vi "turnVelocityPlanning.vi"(4 "v_ang (rad/s)":dbl=4.0 format="%#_13g", 5 "PID gains Angles to turn":T1={"proportional gain (Kc)"=4.0, "integral time (Ti, min)"=0.0, "derivative time (Td, min)"=0.001} {"derivative time (Td, min)" format="%.3f"; "integral time (Ti, min)" format="%.10f"; "proportional gain (Kc)" format="%.3f"}, 6 "radius (mm)":dbl=140.0 format="%.2f", 7 "PID gains radius to turn":T1={"proportional gain (Kc)"=4.0, "integral time (Ti, min)"=0.0, "derivative time (Td, min)"=0.0} {"derivative time (Td, min)" format="%.3f"; "integral time (Ti, min)" format="%.3f"; "proportional gain (Kc)" format="%.3f"}, 8 "error in (no error)":errorcluster, 10 "Clockwise?":bool, 11 "Robot in":refnum<class "Robot.lvclass">) -> (0 "error out":errorcluster, 3 "Robot out":refnum<class "Robot.lvclass">)   [LabVIEW 2023, in "Robot.lvclass"]
uses:
  Robot.lvclass
  C:/Users/ebert/Desktop/roboime/SSL_AI/Object_class/Object.lvclass
  Robot.lvclass/Robot.ctl
  Object_class/Object.lvclass/Object.ctl
  <vilib>/Analysis/coordinate.llb/Wrap Angle (scalar).vi
  <vilib>/Analysis/baseanly.llb/Unit Vector (DBL).vi
  <vilib>/Analysis/coordinate.llb/2D Cartesian Coordinate Rotation (Scalar).vi
  Read dest_x.vi
  Read dest_y.vi
  Object_class/Read position(x,y).vi
  Read orientation.vi
  Write v_ang.vi
  Write v_tang.vi
  Write v_norm.vi
  <vilib>/addons/control/pid/pid.llb/PID (DBL).vi
  <vilib>/Analysis/NI_AALPro.lvlib
  <vilib>/Analysis/NI_AALBase.lvlib
  Utilities_class/Utilities.lvclass
  <vilib>/addons/control/pid/NI_PID_pid.lvlib
  <vilib>/Analysis/NI_AAL_Angle.lvlib
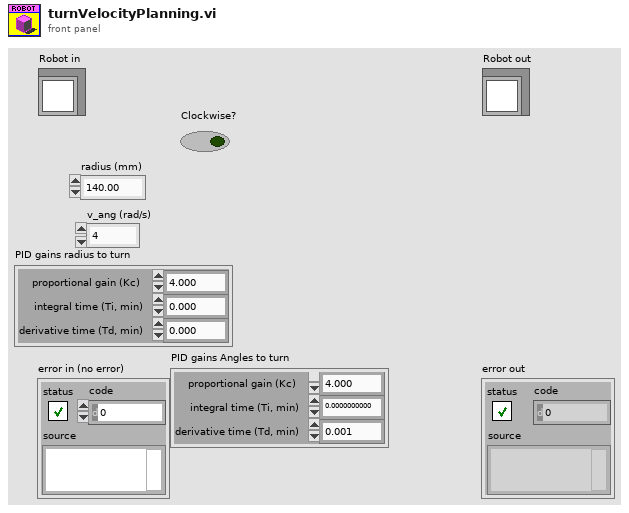
[diagram p1: front panel]
types:
  T1 = cluster{"proportional gain (Kc)":dbl, "integral time (Ti, min)":dbl, "derivative time (Td, min)":dbl}
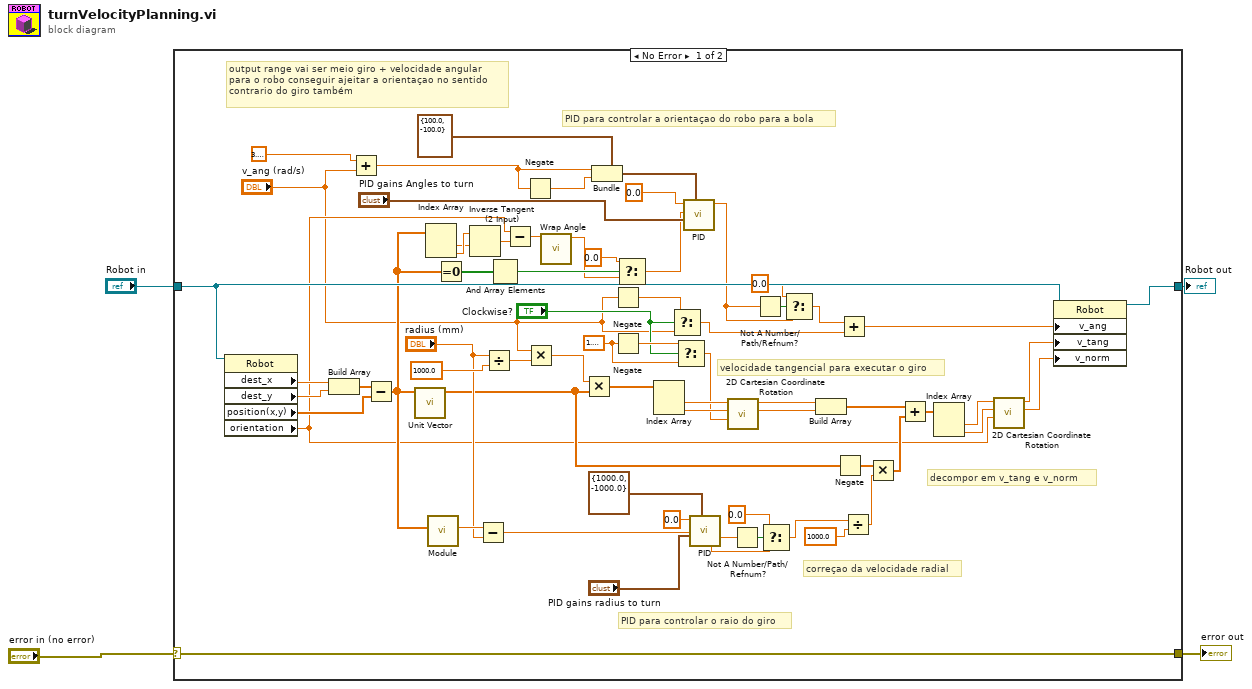
[diagram p0: block diagram]
diagram:
  n1 = case shown="No Error" "error in (no error)" {
    selector: "error in (no error)" -> [w70 w72]
    tunnel: [w70 w72] -> w3
    tunnel: [w61 w71] -> w1
    tunnel: "Robot in" -> [w62 w71]
    frame No Error {
      w27 = 1.5707963267948966
      # "correçao da velocidade radial"
      # "velocidade tangencial para executar o giro"
      # "output range vai ser meio giro + velocidade angular\npara o robo conseguir ajeitar a orientaçao no sentido\ncontrario do giro também"
      # "decompor em v_tang e v_norm"
      # "PID para controlar o raio do giro"
      # "PID para controlar a orientaçao do robo para a bola"
      n2 = property class="Robot"(reference=w62) -> ("dest_x"=w69:dbl, "dest_y"=w68:dbl, "position(x,y)"=w66:dbl[], "orientation"=w19:dbl)  [unwired: 1 in, 2 out]
      n3 = Build Array(w69, w68) -> (w67:dbl[])
      n4 = Add(x=3.141592653589793, y="v_ang (rad/s)") -> (x+y=w15:dbl)
      n5 = Subtract(x=w67, y=w66) -> (x-y=w32:dbl[])
      n6 = call-poly <vilib>:"Unit Vector.vi"("Input Vector"=w32) -> ("Unit Vector"=w43:dbl[])  [unwired: 8 in, 2 out]
      n7 = Index Array(array=w32) -> (element #1=w34:dbl, element #2=w35:dbl)  [unwired: 2 in]
      n8 = call "Module.vi"("2D vector"=w32) -> ("Modulo"=w55:dbl)  [unwired: 8 in, 2 out]
      n9 = Equal To 0?(x=w32) -> (x = 0?=w31:bool[])
      n10 = Inverse Tangent (2 Input)(1:w34, 2:w35) -> (0:w18:dbl)
      n11 = Subtract(x=w55, y="radius (mm)") -> (x-y=w53:dbl)
      n12 = Divide(x="radius (mm)", y=1000.0) -> (x/y=w59:dbl)
      n13 = And Array Elements(Boolean array=w31) -> (logical AND=w30:bool)
      n14 = Subtract(x=w19, y=w18) -> (x-y=w17:dbl)
      n15 = Negate(x=w15) -> (-x=w36:dbl)
      n16 = Multiply(x="v_ang (rad/s)", y=w59) -> (x*y=w58:dbl)
      n17 = call-poly <vilib>:"Wrap Angle.vi"("angle in"=w17) -> ("angle out"=w16:dbl)  [unwired: 9 in, 1 out]
      n18 = Multiply(x=w58, y=w43) -> (x*y=w65:dbl[])
      n19 = Bundle(cluster=cluster{"output high":dbl, "output low":dbl} {"output high"=100.0, "output low"=-100.0} ("output range"), "output high"=w15, "output low"=w36) -> (w37:cluster{"output high":dbl, "output low":dbl})
      n20 = Negate(x="v_ang (rad/s)") -> (-x=w23:dbl)
      n21 = Negate(x=w27) -> (-x=w24:dbl)
      n22 = Select(t=0.0, s=w30, f=w16) -> (s? t:f=w28:dbl)
      n23 = Index Array(array=w65) -> (element #1=w64:dbl, element #2=w63:dbl)  [unwired: 2 in]
      n24 = Select(t=w23, s="Clockwise?", f="v_ang (rad/s)") -> (s? t:f=w25:dbl)
      n25 = Select(t=w24, s="Clockwise?", f=w27) -> (s? t:f=w26:dbl)
      n26 = call-poly <vilib>:"PID.vi"("output range"=w37, "PID gains"="PID gains Angles to turn", "process variable"=w28, "setpoint"=0.0) -> ("output"=w5:dbl)  [unwired: 6 in, 1 out]
      n27 = call-poly <vilib>:"PID.vi"("output range"=cluster{"output high":dbl, "output low":dbl} {"output high"=1000.0, "output low"=-1000.0}, "PID gains"="PID gains radius to turn", "process variable"=w53, "setpoint"=0.0) -> ("output"=w11:dbl)  [unwired: 6 in, 1 out]
      n28 = call-poly <vilib>:"2D Cartesian Coordinate Rotation.vi"("theta"=w26, "y"=w63, "x"=w64) -> ("y out"=w49:dbl, "x out"=w50:dbl)  [unwired: 6 in, 1 out]
      n29 = Not A Number/Path/Refnum?(number/path/refnum=w11) -> (NaN/Path/Refnum?=w12:bool)
      n30 = Not A Number/Path/Refnum?(number/path/refnum=w5) -> (NaN/Path/Refnum?=w7:bool)
      n31 = Select(t=0.0, s=w12, f=w11) -> (s? t:f=w10:dbl)
      n32 = Select(t=0.0, s=w7, f=w5) -> (s? t:f=w6:dbl)
      n33 = Build Array(w50, w49) -> (w48:dbl[])
      n34 = Negate(x=w43) -> (-x=w42:dbl[])
      n35 = Add(x=w6, y=w25) -> (x+y=w33:dbl)
      n36 = Divide(x=w10, y=1000.0) -> (x/y=w41:dbl)
      n37 = Multiply(x=w42, y=w41) -> (x*y=w47:dbl[])
      n38 = Add(x=w48, y=w47) -> (x+y=w46:dbl[])
      n39 = Index Array(array=w46) -> (element #1=w45:dbl, element #2=w44:dbl)  [unwired: 2 in]
      n40 = call-poly <vilib>:"2D Cartesian Coordinate Rotation.vi"("theta"=w19, "y"=w44, "x"=w45) -> ("y out"=w21:dbl, "x out"=w20:dbl)  [unwired: 6 in, 1 out]
      n41 = property class="Robot"(reference=w62, "v_ang"=w33, "v_tang"=w20, "v_norm"=w21) -> (reference out=w61:refnum<class "Robot.lvclass">)  [unwired: 1 in, 1 out]
    }
    frame Error {
    }
  }
  "error out" <- w3
  "Robot out" <- w1
